vi "LED Lights Subsystem.vi"(8 "error in":errorcluster) -> ()   [LabVIEW 2015]
uses:
  <vilib>/Rock Robotics/SystemInterfaces/i2clib/i2c_bus.ctl
  Framework/Robot Global Data.vi
  LED Lights Global.vi
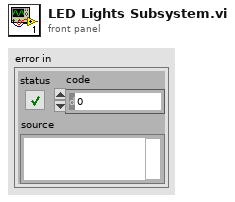
[diagram p1: front panel]
types:
  T1 = typedef "i2c_bus.ctl" = enum16{"I2C On-Board", "I2C MXP", "Invalid"}
  T2 = typedef "LED Lights Ref.ctl" = cluster{"I2CDevRef":T3}
  T3 = typedef "WPI_I2CDevRef.ctl" = cluster{"DevStatus":errorcluster, "Device Address":u8, "Handle":i32, "I2C Bus":T1}
  T4 = typedef "Drive Global Type Def.ctl" = cluster{"Left Drive Motors":T5, "Right Drive Motors":T5}
  T5 = typedef "Master Slave Drive Motors Type Def.ctl" = cluster{"Motor Front":T6, "Motor Back":T6, "Motor Errors":errorcluster, "Motor Top":T6, "Initialized":bool}
  T6 = typedef "Motor Global Type Def.ctl" = cluster{"Motor Error":errorcluster}
  T7 = typedef "NavX Light Global Type Def.ctl" = cluster{"NavX Error":errorcluster, "Initialized":bool}
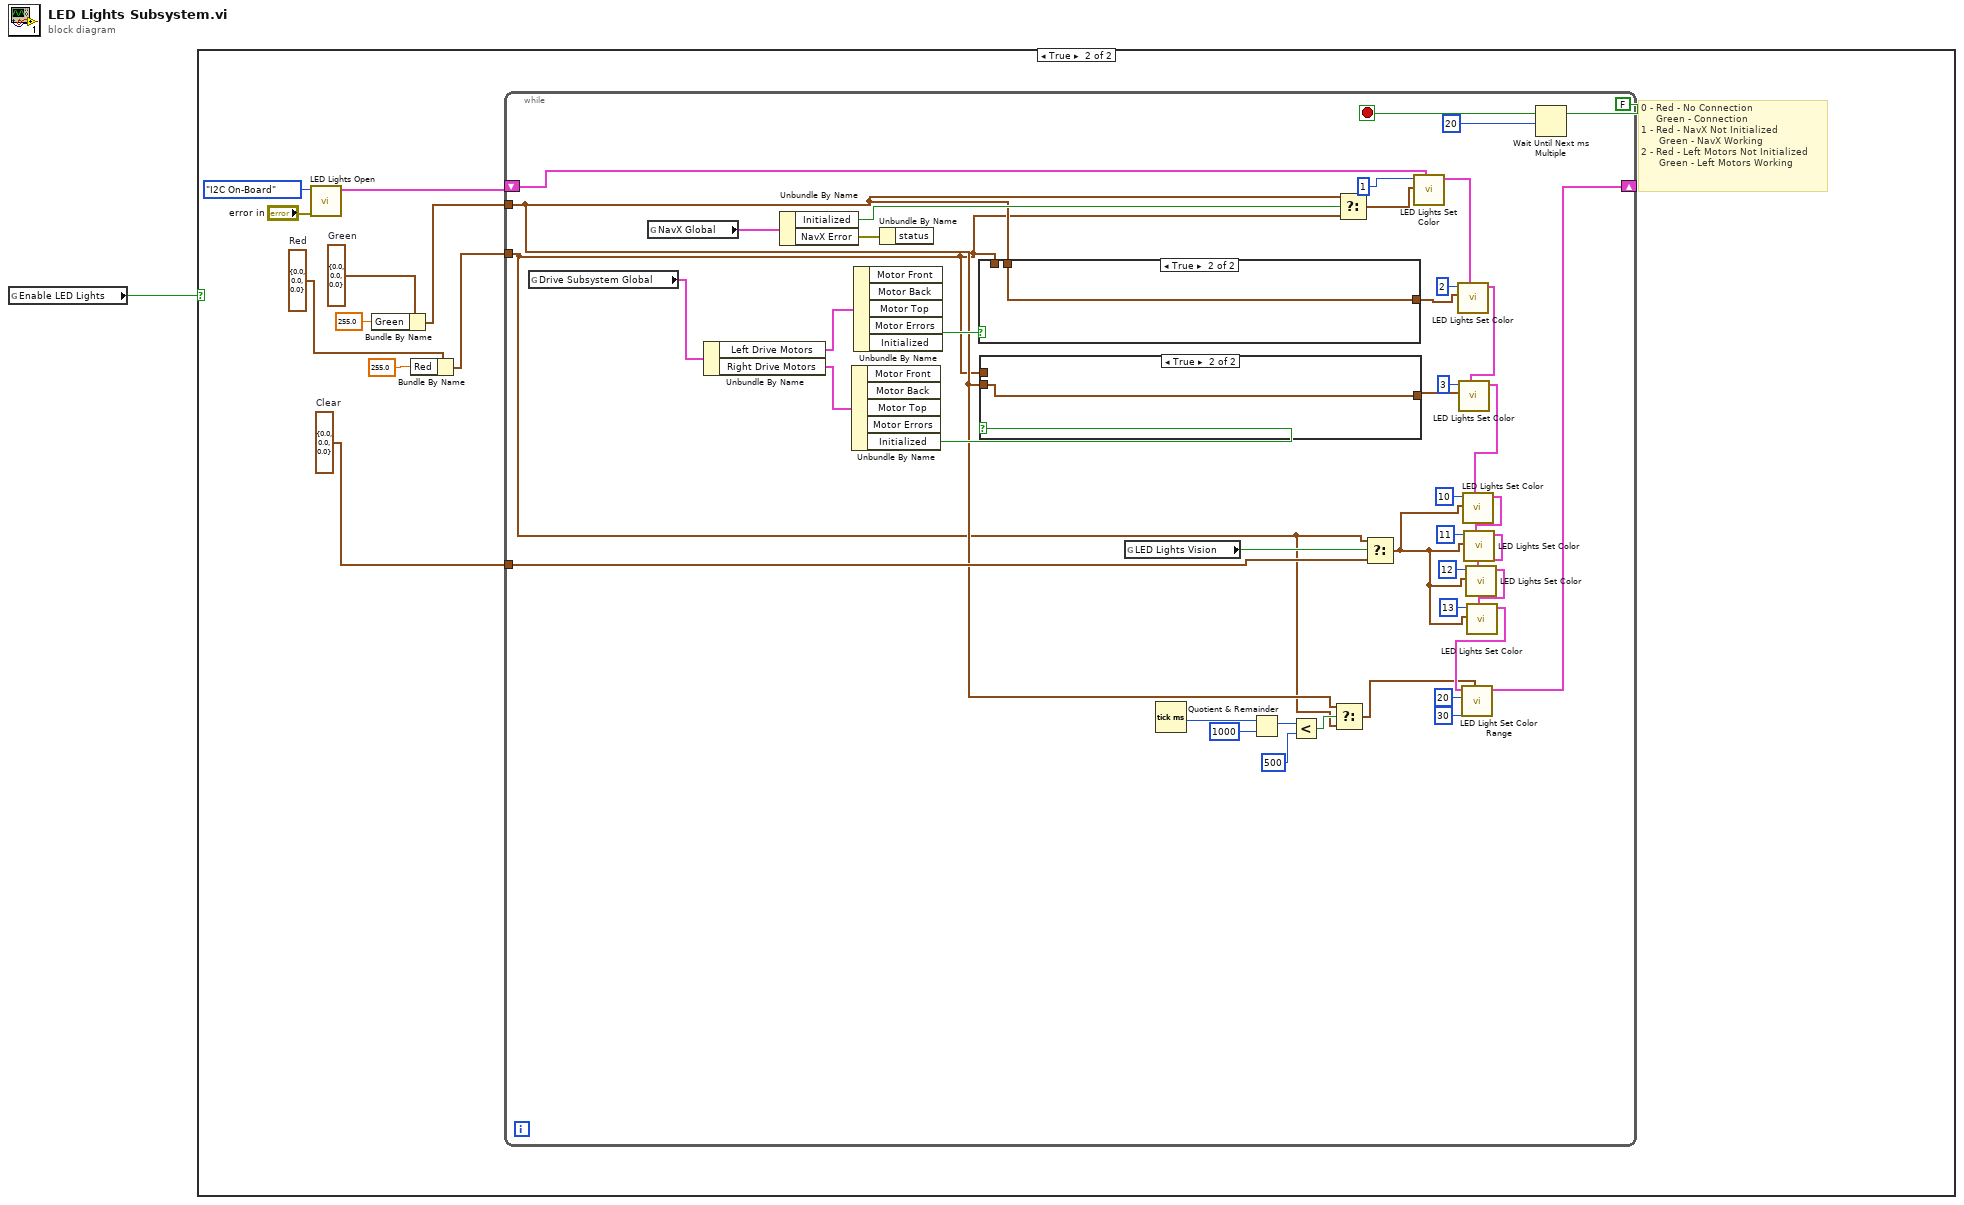
[diagram p0: block diagram]
diagram:
  n1 = global read "Robot Global Data.vi" "Enable LED Lights"() -> (w1:bool)
  n2 = case shown="True" w1 {
    frame False {
    }
    frame True {
      w2 = cluster{"Red":dbl, "Green":dbl, "Blue":dbl} {"Red"=0.0, "Green"=0.0, "Blue"=0.0}  # Clear
      w5 = cluster{"Red":dbl, "Green":dbl, "Blue":dbl} {"Red"=0.0, "Green"=0.0, "Blue"=0.0}  # Red
      w8 = cluster{"Red":dbl, "Green":dbl, "Blue":dbl} {"Red"=0.0, "Green"=0.0, "Blue"=0.0}  # Green
      # "0 - Red - No Connection\n     Green - Connection\n1 - Red - NavX Not Initialized\n      Green - NavX Working\n2 - Red - Left Motors Not Initialized\n      Green - Left Motors Working"
      n3 = call "LED Lights Open.vi"("error in"="error in", "I2C Bus"=i2c_bus."I2C On-Board") -> ("output cluster"=w9:T2)  [unwired: 8 in, 1 out]
      n4 = Bundle By Name(cluster=w8, "Green"=255.0) -> (w6:cluster{"Red":dbl, "Green":dbl, "Blue":dbl})
      n5 = Bundle By Name(cluster=w5, "Red"=255.0 ("Green")) -> (w3:cluster{"Red":dbl, "Green":dbl, "Blue":dbl})
      n6 = while {
        shift-right: [w22] -> _
        shift-left: w9 -> [w50]
        tunnel: w6 -> [w14]
        tunnel: w3 -> [w13]
        tunnel: w2 -> [w27]
        stop <- FALSE stop-if-true
        n7 = global read "LED Lights Global.vi" "Drive Subsystem Global"() -> (w45:T4)
        n8 = global read "LED Lights Global.vi" "NavX Global"() -> (w48:T7)
        n9 = Unbundle By Name(w45) -> ("Left Drive Motors"=w44:T5, "Right Drive Motors"=w43:T5)
        n10 = Unbundle By Name(w48) -> ("Initialized"=w47:bool, "NavX Error"=w51:errorcluster)
        n11 = Unbundle By Name(w43) -> ("Initialized"=w38:bool)  [unwired: 4 out]
        n12 = Unbundle By Name(w44) -> ("Initialized"=w42:bool)  [unwired: 4 out]
        n13 = Unbundle By Name(w51) -> ()  [unwired: 1 out]
        n14 = case shown="True" w42 {
          tunnel: [w56 w57] -> w39
          tunnel: w13 -> [w56 _]
          tunnel: w14 -> [_ w57]
          frame False {
          }
          frame True {
          }
        }
        n15 = case shown="True" w38 {
          tunnel: [w54 w55] -> w36
          tunnel: w13 -> [w54 _]
          tunnel: w14 -> [_ w55]
          frame False {
          }
          frame True {
          }
        }
        n16 = global read "LED Lights Global.vi" "LED Lights Vision"() -> (w28:bool)
        n17 = Tick Count (ms)() -> (millisecond timer value=w19:u32)
        n18 = Quotient & Remainder(x=w19, y=u32 1000) -> (x-y*floor(x/y)=w17:u32)  [unwired: 1 out]
        n19 = Less?(x=w17, y=u32 500) -> (x < y?=w16:bool)
        n20 = Select(t=w14, s=w16, f=w13) -> (s? t:f=w12:cluster{"Red":dbl, "Green":dbl, "Blue":dbl})
        n21 = Select(t=w14, s=w47, f=w13) -> (s? t:f=w46:cluster{"Red":dbl, "Green":dbl, "Blue":dbl})
        n22 = Select(t=w13, s=w28, f=w27) -> (s? t:f=w29:cluster{"Red":dbl, "Green":dbl, "Blue":dbl})
        n23 = call "LED Lights Set Color.vi"("LED Lights Ref In"=w50, "Color"=w46, "Light ID"=u8 1 ("Light ID 2")) -> ("LED Lights Ref Out"=w41:T2)  [unwired: 7 in, 1 out]
        n24 = call "LED Lights Set Color.vi"("LED Lights Ref In"=w41, "Color"=w39, "Light ID"=u8 2) -> ("LED Lights Ref Out"=w37:T2)  [unwired: 7 in, 1 out]
        n25 = call "LED Lights Set Color.vi"("LED Lights Ref In"=w37, "Color"=w36, "Light ID"=u8 3) -> ("LED Lights Ref Out"=w34:T2)  [unwired: 7 in, 1 out]
        n26 = call "LED Lights Set Color.vi"("LED Lights Ref In"=w34, "Color"=w29, "Light ID"=u8 10) -> ("LED Lights Ref Out"=w26:T2)  [unwired: 7 in, 1 out]
        n27 = call "LED Lights Set Color.vi"("LED Lights Ref In"=w26, "Color"=w29, "Light ID"=u8 11) -> ("LED Lights Ref Out"=w25:T2)  [unwired: 7 in, 1 out]
        n28 = call "LED Lights Set Color.vi"("LED Lights Ref In"=w25, "Color"=w29, "Light ID"=u8 12) -> ("LED Lights Ref Out"=w24:T2)  [unwired: 7 in, 1 out]
        n29 = call "LED Lights Set Color.vi"("LED Lights Ref In"=w24, "Color"=w29, "Light ID"=u8 13) -> ("LED Lights Ref Out"=w23:T2)  [unwired: 7 in, 1 out]
        n30 = call "LED Light Set Color Range.vi"("Color"=w12, "Light ID End"=u8 30, "Light ID Start"=u8 20, "LED Lights Ref In"=w23) -> ("LED Lights Ref Out"=w22:T2)  [unwired: 6 in, 1 out]
        n31 = Wait Until Next ms Multiple(millisecond multiple=20) -> ()  [unwired: 1 out]
      }
    }
  }
